vi "Unit test on generation of CRC-16.vi"(2 "Coresponding CRC-16":string[](array[string])=["3798", "41F8", "0CEC", "2ED1", "3278", "3CCD", "2156"], 3 "Cmd or response messages":string[](array[string])=["$TEA,086,040,031,000,", "$TE2", "$PRA,079,000,", "$STA,0301,", "$???,", "$CHP", "$RS1"]) -> (0 "Test results":cluster{"String":string, "Boolean":bool}[](array[cluster]), 1 "Passed":bool)   [LabVIEW 2021, in "F-70 driver.lvlib"]
uses:
  F-70 driver.lvlib
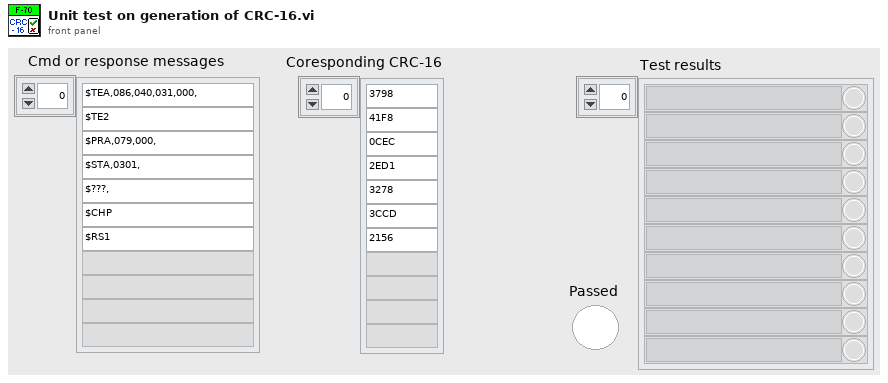
[diagram p1: front panel]
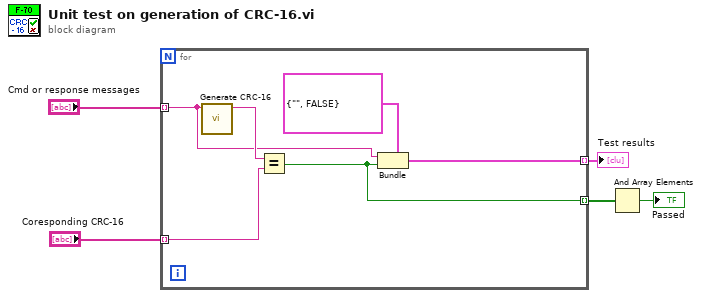
[diagram p0: block diagram]
diagram:
  n1 = for {
    tunnel: "Coresponding CRC-16" -> [w10] mode=indexing
    tunnel: "Cmd or response messages" -> [w7] mode=indexing
    tunnel: [w8] -> w3 mode=indexing
    tunnel: [w6] -> w2 mode=indexing
    n2 = call "Generate CRC-16.vi"("DATA PACKET"=w7) -> ("CRC-16 H-str"=w11:string)  [unwired: 4 in, 2 out]
    n3 = Equal?(x=w11, y=w10) -> (x = y?=w6:bool)
    n4 = Bundle(cluster=cluster{string, bool} {"", FALSE}, w7, w6) -> (w8:cluster{string, bool})
  }
  "Test results" <- w3
  n5 = And Array Elements(Boolean array=w2) -> (logical AND=→"Passed":bool)
